vi "upload.vi"(8 "error in (no error)":errorcluster, 11 "CameraControlViewer in":refnum<class "CameraControlViewer.lvclass">) -> (0 "error out":errorcluster, 3 "CameraControlViewer out":refnum<class "CameraControlViewer.lvclass">)   [LabVIEW 2009, in "Views.lvlib" / "Camera.lvlib" / "CameraControlViewer.lvclass"]
uses:
  CameraControlViewer.lvclass
  Tools/CameraSettings/PixelFlySettings/PixelflySettings.lvclass
  Tools/Filing/FileSystem/FileSystem.lvclass
  Tools/Settings.lvlib
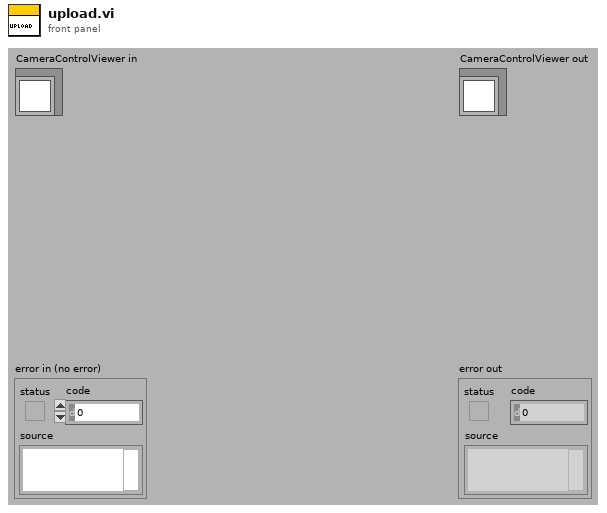
[diagram p1: front panel]
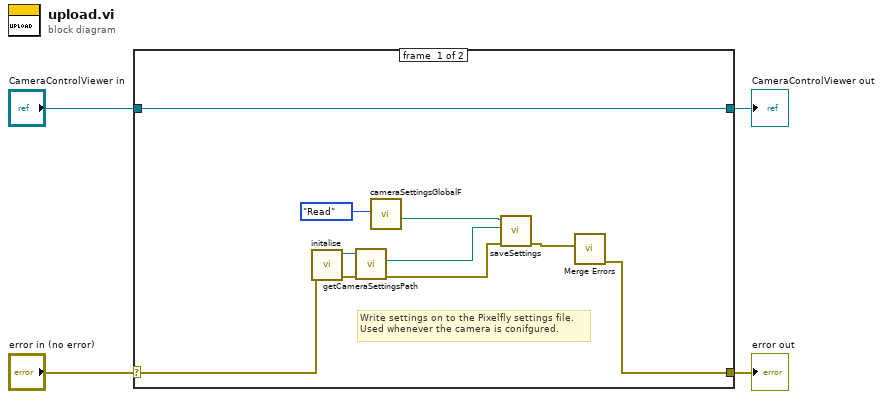
[diagram p0: block diagram]
diagram:
  n1 = case shown="No Error" "error in (no error)" {
    selector: "error in (no error)" -> [w10 w16]
    tunnel: [w8 w16] -> w3
    tunnel: [w7 w15] -> w1
    tunnel: "CameraControlViewer in" -> [w7 w15]
    frame #0 {
      # "Write settings on to the Pixelfly settings file.\nUsed whenever the camera is conifgured."
      n2 = call "initalise.vi"("error in (no error)"=w10) -> ("error out"=w11:errorcluster, "FileSystem out"=w13:refnum<class "FileSystem.lvclass">)  [unwired: 9 in]
      n3 = call-dynamic "getCameraSettingsPath.vi"("error in (no error)"=w11, "FileSystem.lvclass in"=w13) -> ("error out"=w5:errorcluster, "CameraSettingsPath"=w12:path)  [unwired: 7 in, 1 out]
      n4 = call "cameraSettingsGlobalF.vi"("Action"=enum16{"Write", "Read"}."Read") -> ("PixelflySettings"=w6:refnum<class "PixelflySettings.lvclass">)  [unwired: 10 in]
      n5 = call-dynamic "saveSettings.vi"("error in (no error)"=w5, "Path"=w12, "PixelflySettings in"=w6) -> ("error out"=w9:errorcluster)  [unwired: 7 in, 1 out]
      n6 = call <vilib>:"Merge Errors.vi"("error in 2 (no error)"=w9) -> ("error out"=w8:errorcluster)  [unwired: 6 in]
    }
    frame #1 {
    }
  }
  "error out" <- w3
  "CameraControlViewer out" <- w1
